vi "CS580_SetCurent_DC.vi"(8 "error in":errorcluster, 10 "Current (A)":dbl, 11 "VISA Refnum in":refnum<visa-resource-name>) -> (0 "error out":errorcluster, 3 "VISA resource name out":refnum<visa-resource-name>)   [LabVIEW 2023]
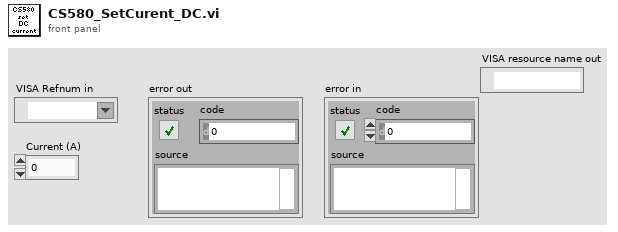
[diagram p1: front panel]
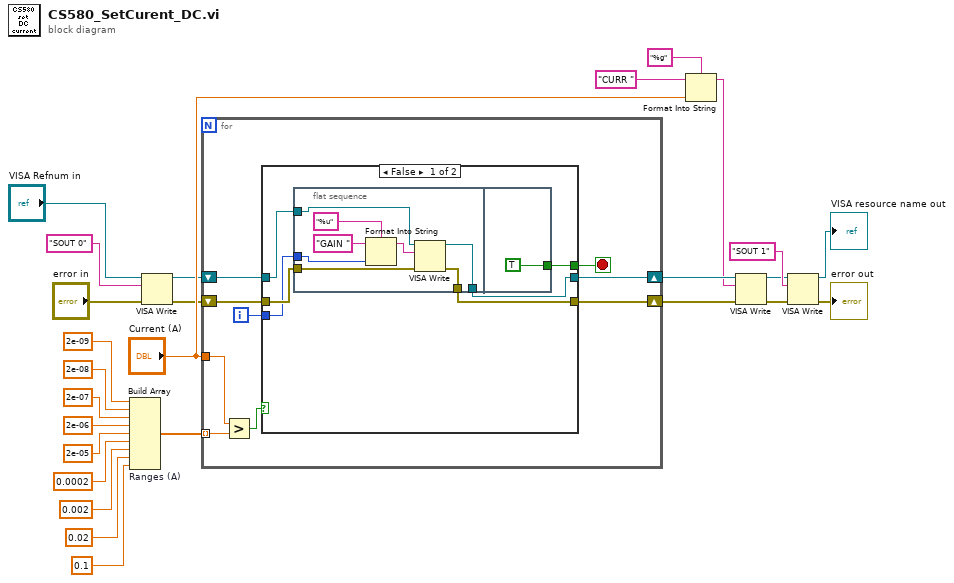
[diagram p0: block diagram]
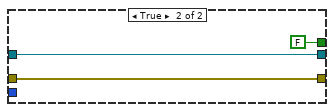
[diagram p2: hidden frame]
diagram:
  n1 = Build Array "Ranges (A)"(2e-09 ("element"), 2e-08 ("element"), 2e-07 ("element"), 2e-06 ("element"), 2e-05 ("element"), 0.0002 ("element"), 0.002 ("element"), 0.02 ("element"), 0.1 ("element")) -> (w25:dbl[])
  n2 = VISA Write(VISA resource name="VISA Refnum in", write buffer="SOUT 0", error in (no error)="error in") -> (VISA resource name out=w20:refnum<visa-resource-name>, error out=w21:errorcluster)  [unwired: 1 out]
  n3 = for {
    tunnel: w25 -> [w35] mode=indexing
    shift-right: [w29] -> w17
    shift-left: w20 -> [w33]
    shift-right: [w28] -> w18
    shift-left: w21 -> [w32]
    tunnel: "Current (A)" -> [w27]
    i -> [w31]
    stop <- w30 stop-if-true
    n4 = Greater?(x=w27, y=w35) -> (0:w34:bool)
    n5 = case shown="False" w34 {
      tunnel: w33 -> [w41 w53]
      tunnel: w32 -> [w40 w52]
      tunnel: w31 -> [w39 _]
      tunnel: [w38 FALSE] -> w30
      tunnel: [w37 w53] -> w29
      tunnel: [w36 w52] -> w28
      frame False {
        n6 = flat-sequence {
          tunnel: w41 -> [w49]
          tunnel: w40 -> [w48]
          tunnel: w39 -> [w45]
          tunnel: [w43] -> w37
          tunnel: [w42] -> w36
          tunnel: [TRUE] -> w38
          frame #0 {
            n7 = Format Into String(format string="%u", initial string="GAIN ", w45) -> (resulting string=w44:string)  [unwired: 1 in, 1 out]
            n8 = VISA Write(VISA resource name=w49, write buffer=w44, error in (no error)=w48) -> (VISA resource name out=w43:refnum<visa-resource-name>, error out=w42:errorcluster)  [unwired: 1 out]
          }
          frame #1 {
          }
        }
      }
      frame True {
      }
    }
  }
  n9 = Format Into String(format string="%g", initial string="CURR ", "Current (A)") -> (resulting string=w7:string)  [unwired: 1 in, 1 out]
  n10 = VISA Write(VISA resource name=w17, write buffer=w7, error in (no error)=w18) -> (VISA resource name out=w22:refnum<visa-resource-name>, error out=w23:errorcluster)  [unwired: 1 out]
  n11 = VISA Write(VISA resource name=w22, write buffer="SOUT 1", error in (no error)=w23) -> (VISA resource name out=→"VISA resource name out":refnum<visa-resource-name>, error out=→"error out":errorcluster)  [unwired: 1 out]
